vi "Check_with_Jump.vi"(4 "Rotation (deg)":dbl format="%#.2f", 5 "Simulate/Run":T1=enum."Run VI", 6 "Exclude Array":T2[](array[typedef])=[{"Sizes"=[{"Max"=1000.0, "Min"=-1000.0}, {"Max"=1000.0, "Min"=-1000.0}, {"Max"=20.0, "Min"=0.0}], "Name"="Roughness Elements", "Exclude Type"=enum."Allow only vertical moves"}, {"Sizes"=[{"Max"=50.0, "Min"=-50.0}, {"Max"=50.0, "Min"=-50.0}, {"Max"=220.0, "Min"=-0.0}], "Name"="B204", "Exclude Type"=enum."Exclude completely"}] {"Sizes"."Min" format="%#.1f"; "Sizes"."Max" format="%#.1f"}, 7 "Traverse Name":string, 8 "Probe Volume":T3=[{"Max"=10.0, "Min"=-10.0}, {"Max"=10.0, "Min"=-10.0}, {"Max"=200.0, "Min"=0.0}] {"Min" format="%#.1f"; "Max" format="%#.1f"}, 9 "Entire Space":T3=[{"Max"=500.0, "Min"=-500.0}, {"Max"=1000.0, "Min"=-1000.0}, {"Max"=700.0, "Min"=0.0}] {"Min" format="%#.1f"; "Max" format="%#.1f"}, 10 "New Position":dbl[](array[numeric])=[0.0, 100.0, 40.0] format="%.2f", 11 "Current position":dbl[](array[numeric])=[0.0, 200.0, 40.0] format="%.2f") -> (1 "Steps":dbl[][](array[numeric])=[[0.0, 200.0, 40.0]] format="%.2f", 3 "Error Comments":string)   [LabVIEW 2010]
uses:
  Box_size.ctl
  Exclude_cluster.ctl
  Exclusion_type.ctl
  Controls/User_Specific_mode.ctl
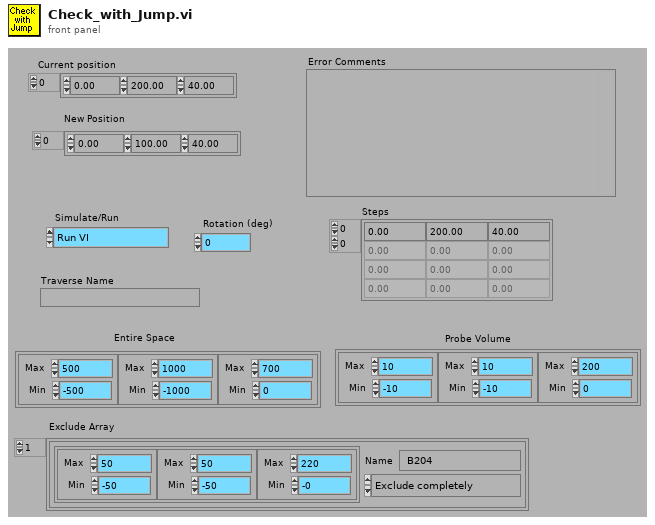
[diagram p1: front panel]
types:
  T1 = typedef "User_Specific_mode.ctl" = enum16{"Check VI only", "Run VI"}
  T2 = typedef "Exclude_cluster.ctl" = cluster{"Sizes":T3, "Name":string, "Exclude Type":T4}
  T3 = typedef "Box_size.ctl" = cluster{"Max":dbl, "Min":dbl}[]
  T4 = typedef "Exclusion_type.ctl" = enum16{"Exclude completely", "Allow only vertical moves"}
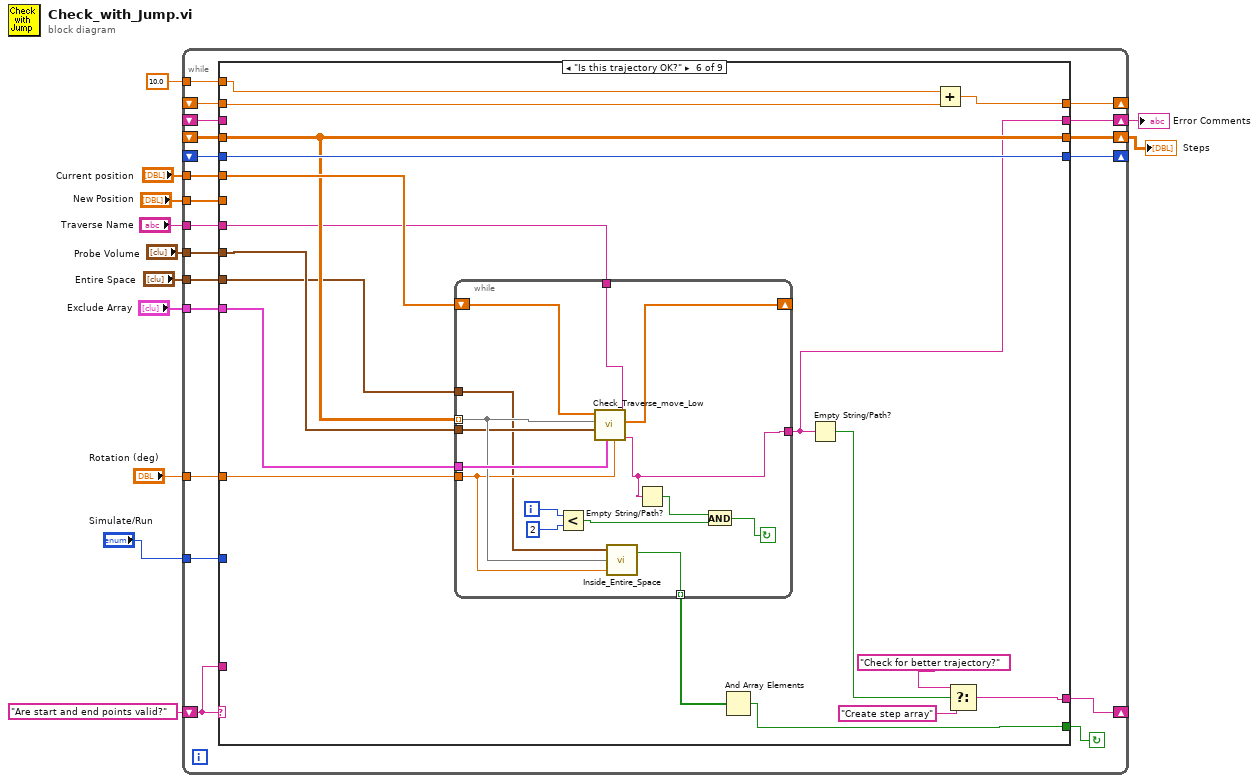
[diagram p0: block diagram]
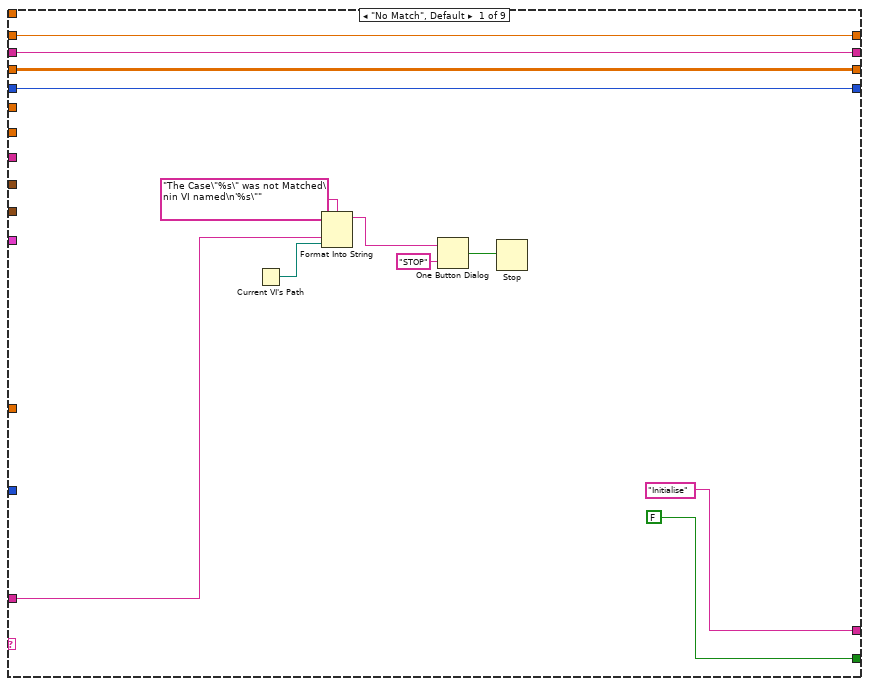
[diagram p2: hidden frame]
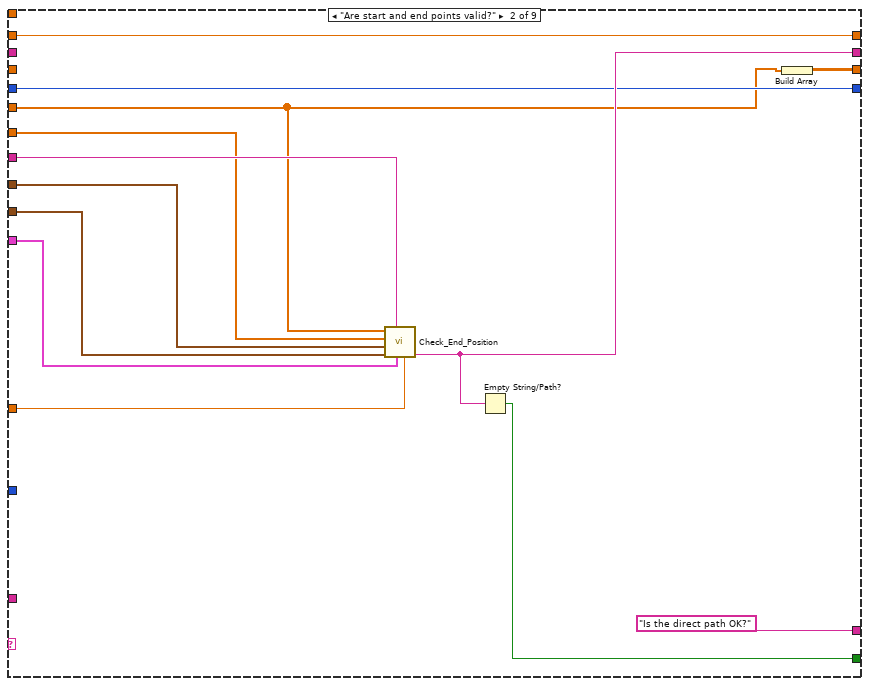
[diagram p3: hidden frame]
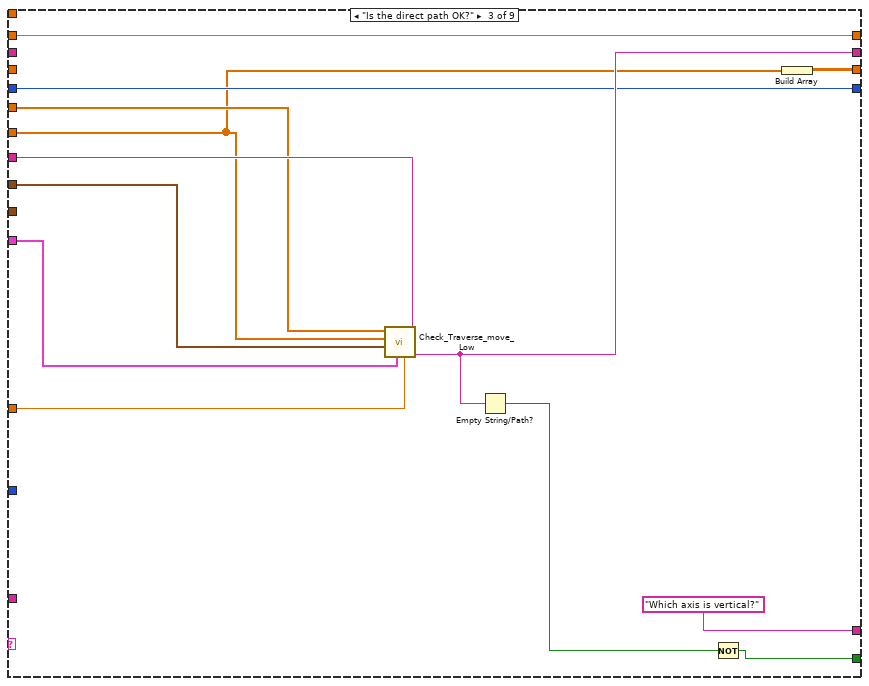
[diagram p4: hidden frame]
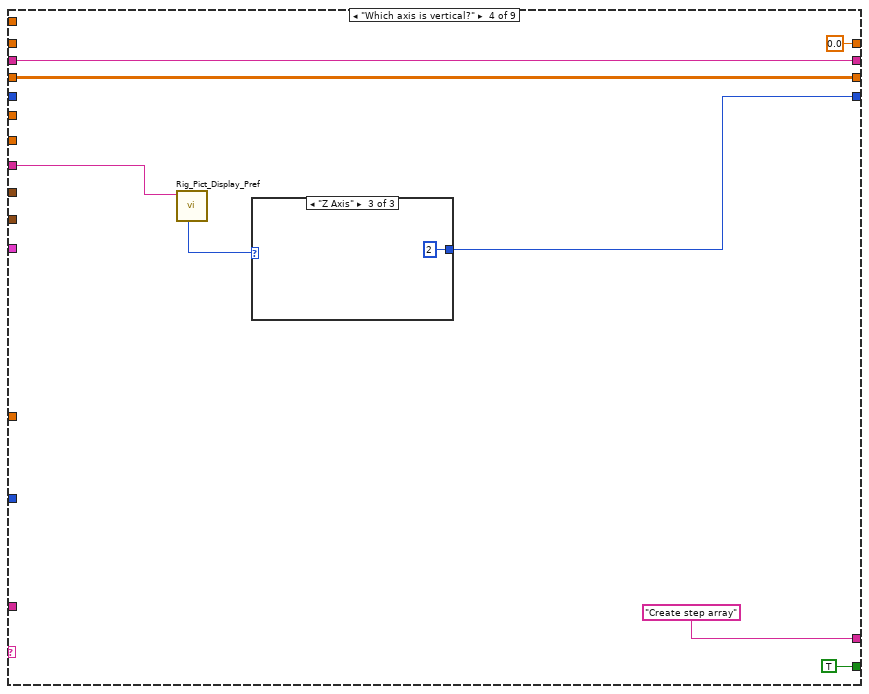
[diagram p5: hidden frame]
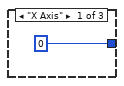
[diagram p6: hidden frame]
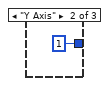
[diagram p7: hidden frame]
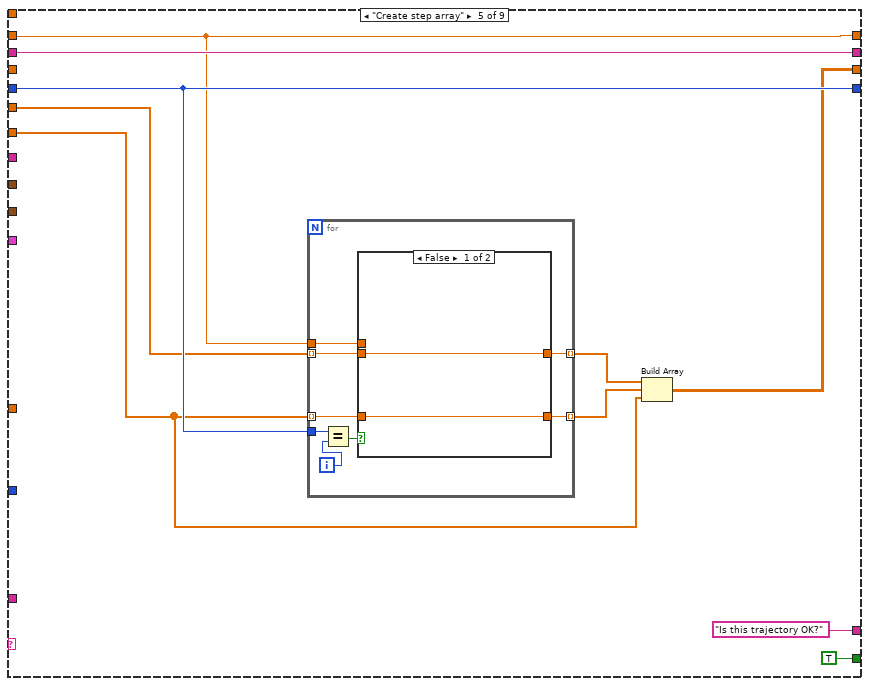
[diagram p8: hidden frame]
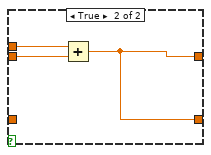
[diagram p9: hidden frame]
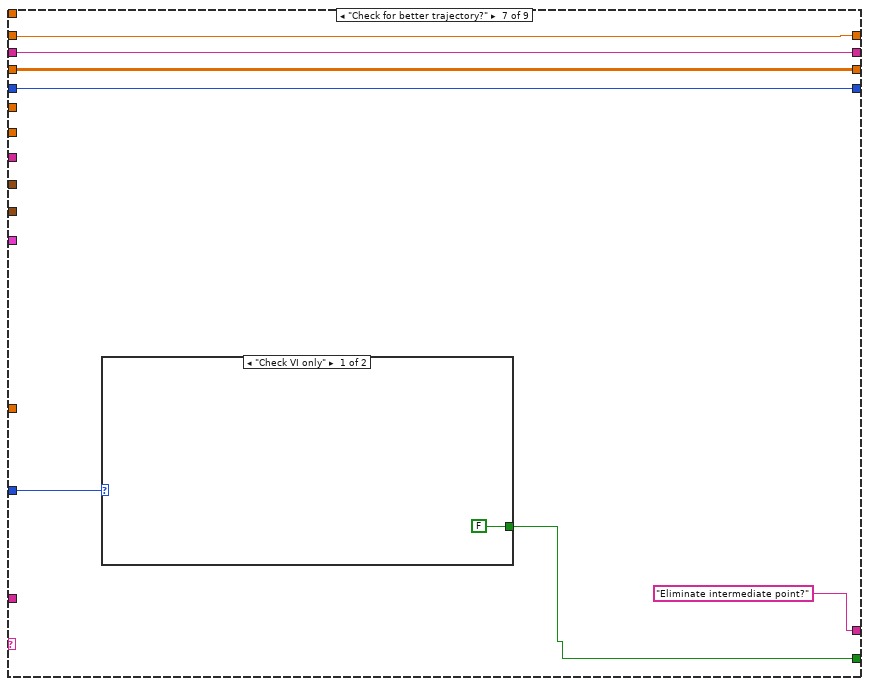
[diagram p10: hidden frame]
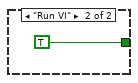
[diagram p11: hidden frame]
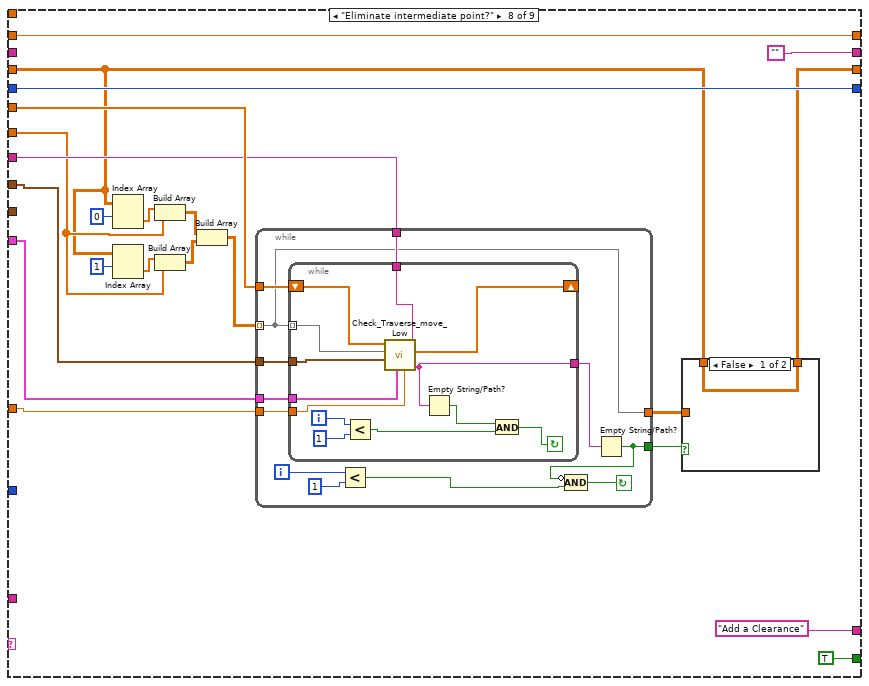
[diagram p12: hidden frame]
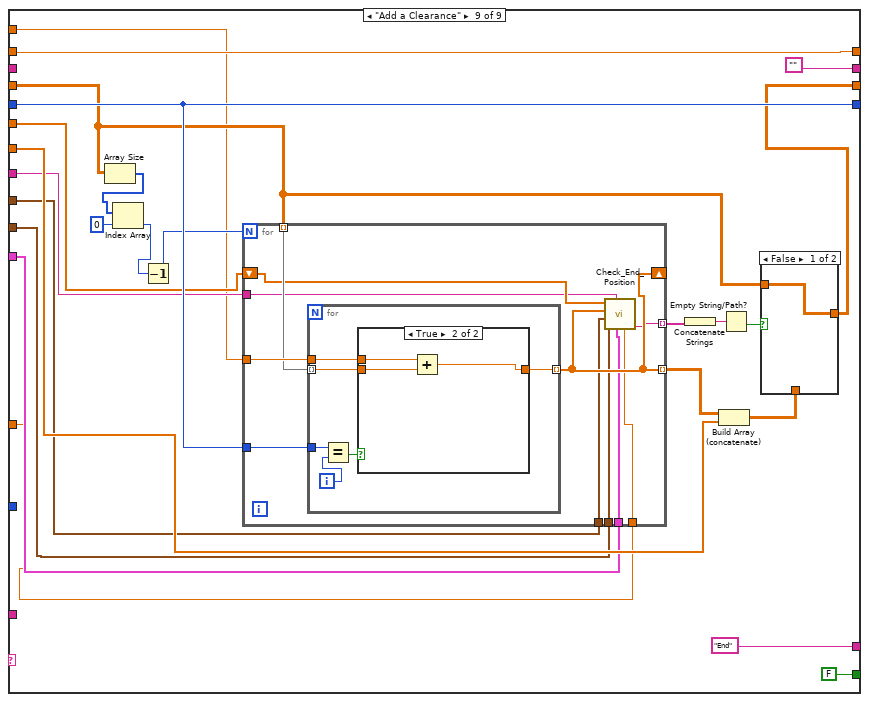
[diagram p14: hidden frame]
diagram:
  n1 = while {
    shift-left: "Are start and end points valid?" -> [w31]
    shift-right: [w32] -> _
    shift-right: [w28] -> w4
    shift-left: _ -> [w29]
    shift-right: [w27] -> w5
    shift-left: _ -> [w26]
    tunnel: "Current position" -> [w25]
    tunnel: "New Position" -> [w24]
    tunnel: "Probe Volume" -> [w23]
    tunnel: "Entire Space" -> [w22]
    tunnel: "Exclude Array" -> [w21]
    tunnel: "Traverse Name" -> [w20]
    shift-right: [w19] -> _
    shift-left: _ -> [w18]
    shift-right: [w17] -> _
    shift-left: _ -> [w16]
    tunnel: 10.0 -> [w15]
    tunnel: "Simulate/Run" -> [w14]
    tunnel: "Rotation (deg)" -> [w13]
    stop <- w30 continue-if-true
    n2 = case shown="\"Is this trajectory OK?\"" w31 {
      tunnel: [FALSE w50 w62 TRUE TRUE w105 w138 TRUE FALSE] -> w30
      tunnel: ["Initialise" "Is the direct path OK?" "Which axis is vertical?" "Create step array" "Is this trajectory OK?" w115 "Eliminate intermediate point?" "Add a Clearance" "End"] -> w32
      tunnel: w31 -> [w39 _ _ _ _ _ _ _ _]
      tunnel: w29 -> [w36 _ _ w76 w90 _ w144 _ _]
      tunnel: [w36 w52 w66 w76 w90 w112 w144 "" ""] -> w28
      tunnel: [w35 w51 w64 w77 w83 w120 w141 w154 w204] -> w27
      tunnel: w26 -> [w35 _ _ w77 _ w120 w141 w152 w203]
      tunnel: w25 -> [_ w46 w65 _ w87 w121 _ w167 w209]
      tunnel: w24 -> [_ w47 w59 _ w84 _ _ w159 w210]
      tunnel: w23 -> [_ w56 w69 _ _ w119 _ w166 w202]
      tunnel: w22 -> [_ w55 _ _ _ w107 _ _ w201]
      tunnel: w21 -> [_ w54 w68 _ _ w118 _ w165 w200]
      tunnel: w20 -> [_ w53 w67 w75 _ w117 _ w164 w199]
      tunnel: [w34 w49 w61 w73 w88 w122 w143 w168 w217] -> w19
      tunnel: w18 -> [w34 w49 w61 _ w88 w122 w143 w168 w217]
      tunnel: [w33 w48 w60 0.0 w82 w109 w142 w151 w215] -> w17
      tunnel: w16 -> [w33 w48 w60 _ w82 w111 w142 w151 w215]
      tunnel: w15 -> [_ _ _ _ _ w110 _ _ w197]
      tunnel: w14 -> [_ _ _ _ _ _ w140 _ _]
      tunnel: w13 -> [_ w45 w58 _ _ w108 _ w147 w196]
      frame "No Match", Default {
        n3 = Current VI's Path() -> (path=w38:path)
        n4 = Format Into String(format string="The Case\"%s\" was not Matched\nin VI named\n'%s\"" ("Format String"), w39, w38) -> (resulting string=w42:string)  [unwired: 2 in, 1 out]
        n5 = One Button Dialog(message=w42, button name ("OK")="STOP") -> (true=w40:bool)
        n6 = Stop(stop? (T)=w40) -> ()
      }
      frame "Are start and end points valid?" {
        n7 = call "Check_End_Position.vi"("Rotation (deg)"=w45, "Exclude Array"=w54, "Traverse Name"=w53, "Entire Space"=w55, "Probe Volume"=w56, "New Position"=w47, "Current position"=w46) -> ("Error Comments"=w52:string)  [unwired: 3 out]
        n8 = Empty String/Path?(string/path=w52) -> (empty?=w50:bool)
        n9 = Build Array(w46) -> (w51:dbl[][])
      }
      frame "Is the direct path OK?" {
        n10 = call "Check_Traverse_move_Low.vi"("Traverse Name"=w67, "Rotation (deg)"=w58, "Exclude Array"=w68, "Probe Volume"=w69, "New Position"=w59, "Current position"=w65) -> ("Error Comments"=w66:string)  [unwired: 3 out]
        n11 = Empty String/Path?(string/path=w66) -> (empty?=w63:bool)
        n12 = Not(x=w63) -> (.not. x?=w62:bool)
        n13 = Build Array(w59) -> (w64:dbl[][])
      }
      frame "Which axis is vertical?" {
        n14 = call "Rig_Pict_Display_Pref.vi"("Traverse Name"=w75) -> ("Which Axis is vertical?"=w74:enum16{"X Axis", "Y Axis", "Z Axis"})  [unwired: 7 out]
        n15 = case shown="\"Z Axis\"" w74 {
          tunnel: [0 1 2] -> w73
          frame "X Axis" {
          }
          frame "Y Axis" {
          }
          frame "Z Axis" {
          }
        }
      }
      frame "Create step array" {
        n16 = for {
          tunnel: w82 -> [w99]
          tunnel: w88 -> [w96]
          tunnel: w87 -> [w95] mode=indexing
          tunnel: [w94] -> w86 mode=indexing
          tunnel: w84 -> [w93] mode=indexing
          tunnel: [w92] -> w85 mode=indexing
          i -> [w98]
          n17 = Equal?(x=w96, y=w98) -> (x = y?=w97:bool)
          n18 = case shown="False" w97 {
            tunnel: w99 -> [_ w104]
            tunnel: w95 -> [w101 w103]
            tunnel: [w101 w102] -> w94
            tunnel: w93 -> [w100 _]
            tunnel: [w100 w102] -> w92
            frame False {
            }
            frame True {
              n19 = Add(x=w104, y=w103) -> (x+y=w102:dbl)
            }
          }
        }
        n20 = Build Array(w86, w85, w84) -> (w83:dbl[][])
      }
      frame "Is this trajectory OK?" {
        n21 = while {
          shift-right: [w131] -> _
          shift-left: w121 -> [w132]
          tunnel: w120 -> [w127] mode=indexing
          tunnel: w119 -> [w126]
          tunnel: w118 -> [w129]
          tunnel: w117 -> [w130]
          tunnel: [w128] -> w112
          tunnel: w108 -> [w125]
          tunnel: w107 -> [w123]
          tunnel: [w124] -> w106 mode=indexing
          i -> [w133]
          stop <- w134 continue-if-true
          n22 = Less?(x=w133, y=2 ("x")) -> (x < y?=w135:bool)
          n23 = call "Check_Traverse_move_Low.vi"("Traverse Name"=w130, "Rotation (deg)"=w125, "Exclude Array"=w129, "Probe Volume"=w126, "New Position"=w127, "Current position"=w132) -> ("Error Comments"=w128:string, "Position At Crash"=w131:dbl[])  [unwired: 2 out]
          n24 = call "Inside_Entire_Space.vi"("Rotation (deg)"=w125, "Current Position"=w127, "Envelope"=w123) -> ("Box Inside"=w124:bool)  [unwired: 1 out]
          n25 = Empty String/Path?(string/path=w128) -> (empty?=w136:bool)
          n26 = And(x=w136, y=w135) -> (x .and. y?=w134:bool)
        }
        n27 = And Array Elements(Boolean array=w106) -> (logical AND=w105:bool)
        n28 = Empty String/Path?(string/path=w112) -> (empty?=w116:bool)
        n29 = Add(x=w110, y=w111) -> (x+y=w109:dbl)
        n30 = Select(t="Check for better trajectory?", s=w116, f="Create step array") -> (s? t:f=w115:string)
      }
      frame "Check for better trajectory?" {
        n31 = case shown="\"Check VI only\"" w140 {
          tunnel: [FALSE TRUE] -> w138
          frame "Check VI only" {
          }
          frame "Run VI" {
          }
        }
      }
      frame "Eliminate intermediate point?" {
        n32 = Index Array(array=w152, index (row)=0) -> (element=w161:dbl[])  [unwired: 1 in]
        n33 = Index Array(array=w152, index (row)=1) -> (element=w160:dbl[])  [unwired: 1 in]
        n34 = Build Array(w161, w159) -> (w158:dbl[][])
        n35 = Build Array(w160, w159) -> (w157:dbl[][])
        n36 = Build Array(w158, w157) -> (w156:dbl[][][])
        n37 = while {
          tunnel: w167 -> [w182]
          tunnel: w166 -> [w181]
          tunnel: w165 -> [w180]
          tunnel: w164 -> [w179]
          tunnel: w156 -> [w172] mode=indexing
          tunnel: [w173] -> w155
          tunnel: [w172] -> w153
          tunnel: w147 -> [w171]
          i -> [w176]
          stop <- w174 continue-if-true
          n38 = while {
            shift-right: [w191] -> _
            shift-left: w182 -> [w195]
            tunnel: w181 -> [w194]
            tunnel: w180 -> [w193]
            tunnel: w179 -> [w192]
            tunnel: [w185] -> w178
            tunnel: w172 -> [w184] mode=indexing
            tunnel: w171 -> [w183]
            i -> [w190]
            stop <- w186 continue-if-true
            n39 = Less?(x=w190, y=1 ("x")) -> (x < y?=w187:bool)
            n40 = call "Check_Traverse_move_Low.vi"("Traverse Name"=w192, "Rotation (deg)"=w183, "Exclude Array"=w193, "Probe Volume"=w194, "New Position"=w184, "Current position"=w195) -> ("Error Comments"=w185:string, "Position At Crash"=w191:dbl[])  [unwired: 2 out]
            n41 = Empty String/Path?(string/path=w185) -> (empty?=w188:bool)
            n42 = And(x=w188, y=w187) -> (x .and. y?=w186:bool)
          }
          n43 = Less?(x=w176, y=1 ("x")) -> (x < y?=w175:bool)
          n44 = Empty String/Path?(string/path=w178) -> (empty?=w173:bool)
          n45 = Compound Arithmetic op=AND(invert w173, w175) -> (w174:bool)
        }
        n46 = case shown="False" w155 {
          tunnel: [w169 w170] -> w154
          tunnel: w153 -> [_ w170]
          tunnel: w152 -> [w169 _]
          frame False {
          }
          frame True {
          }
        }
      }
      frame "Add a Clearance" {
        n47 = Array Size(array=w203) -> (size(s)=w214:i32[])
        n48 = Index Array(array=w214, index=0) -> (element=w212:i32)
        n49 = Decrement(x=w212) -> (x-1=w211:i32)
        n50 = for {
          N: w211 -> [_]
          tunnel: w217 -> [w232]
          tunnel: [w228] -> w216 mode=indexing
          tunnel: w197 -> [w231]
          tunnel: w203 -> [w230] mode=indexing
          shift-right: [w228] -> _
          shift-left: w209 -> [w229]
          tunnel: [w227] -> w208 mode=indexing
          tunnel: w202 -> [w226]
          tunnel: w201 -> [w225]
          tunnel: w200 -> [w224]
          tunnel: w199 -> [w223]
          tunnel: w196 -> [w222]
          n51 = for {
            tunnel: w231 -> [w238]
            tunnel: w232 -> [w235]
            tunnel: w230 -> [w234] mode=indexing
            tunnel: [w233] -> w228 mode=indexing
            i -> [w237]
            n52 = Equal?(x=w235, y=w237) -> (x = y?=w236:bool)
            n53 = case shown="True" w236 {
              tunnel: w238 -> [_ w242]
              tunnel: w234 -> [w239 w241]
              tunnel: [w239 w240] -> w233
              frame False {
              }
              frame True {
                n54 = Add(x=w242, y=w241) -> (x+y=w240:dbl)
              }
            }
          }
          n55 = call "Check_End_Position.vi"("Rotation (deg)"=w222, "Exclude Array"=w224, "Traverse Name"=w223, "Entire Space"=w225, "Probe Volume"=w226, "New Position"=w228, "Current position"=w229) -> ("Error Comments"=w227:string)  [unwired: 3 out]
        }
        n56 = Concatenate Strings(w208) -> (w207:string)
        n57 = Build Array (concatenate)(w216, w210) -> (w205:dbl[][])
        n58 = Empty String/Path?(string/path=w207) -> (empty?=w206:bool)
        n59 = case shown="False" w206 {
          tunnel: w205 -> [_ w221]
          tunnel: [w220 w221] -> w204
          tunnel: w203 -> [w220 _]
          frame False {
          }
          frame True {
          }
        }
      }
    }
  }
  "Error Comments" <- w4
  "Steps" <- w5
